vi "Highlight.vi"() -> ()   [LabVIEW 2017]
uses:
  <vilib>/Utility/traverseref.llb/TRef TravTarget.ctl
  user.lib/_NEVSTOP/Communicable State Machine(CSM)/_Polymophic/Add State(s) to Queue By BOOL(Element).vi
  user.lib/_NEVSTOP/Communicable State Machine(CSM)/Communicable State Machine.lvlib
  <vilib>/Utility/traverseref.llb/VI Scripting - Traverse.lvlib
panel:
  in  "Highlight All Scripts":bool
  in  "Highlight Scripts":bool
  out "String":string
  in  "Listbox":i32(listbox)
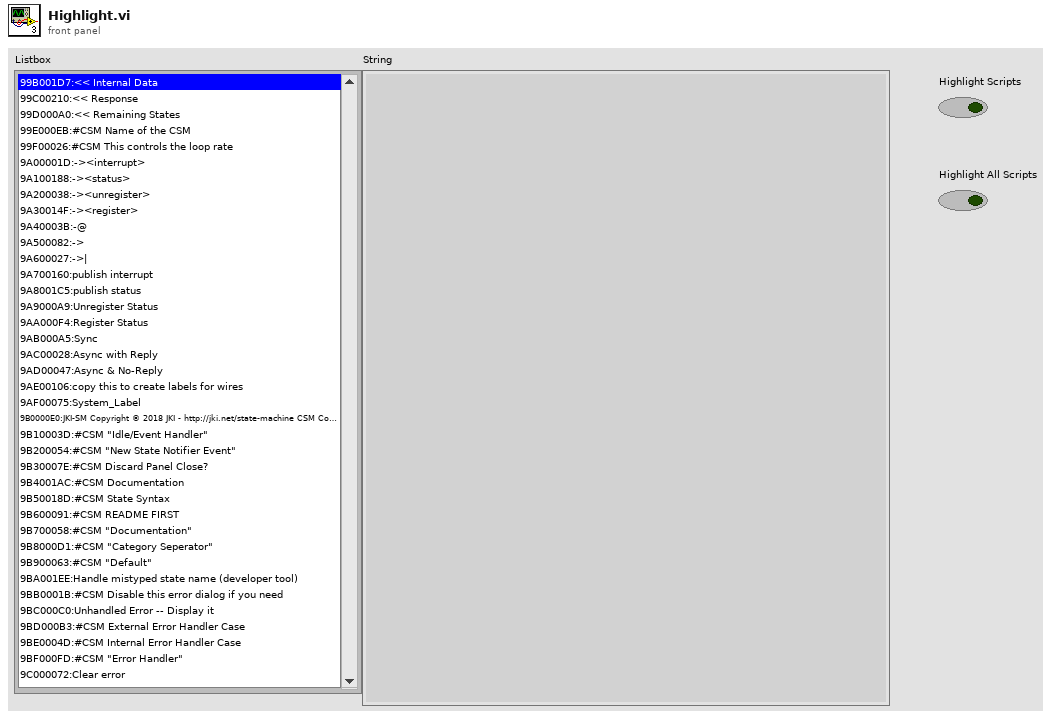
[diagram p1: front panel]
types:
  T1 = enum32{"Invalid", "Standard", "Closed", "Hidden", "Minimized", "Maximized"}
  T2 = enum32{"invalid app kind", "Development System", "Run Time System", "Student Edition", "Embedded LabVIEW", "Evaluation", "Custom"}
  T3 = typedef "TRef TravTarget.ctl" = enum16{"FP", "BD", "Other"}
  T4 = cluster{"Core":cluster{"Current VI Reference":refnum<vi>, "Close Panel on Exit?":bool}, "VI":path, "VIRef":refnum<vi>}
  T5 = cluster{"Current VI Reference":refnum<vi>, "Close Panel on Exit?":bool}
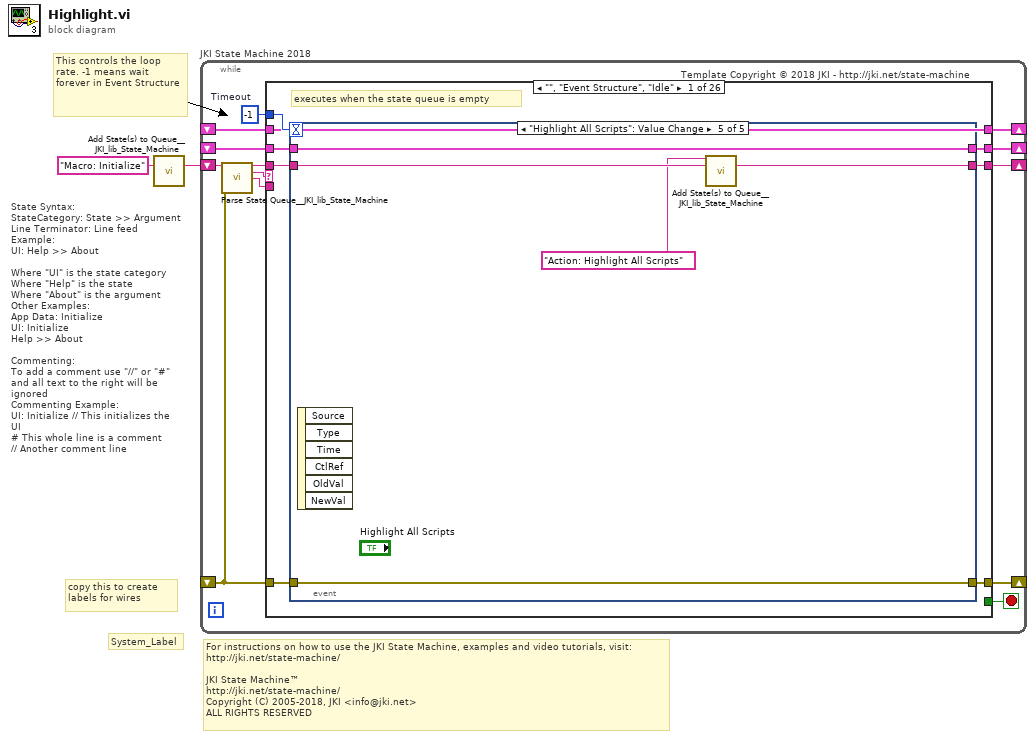
[diagram p0: block diagram]
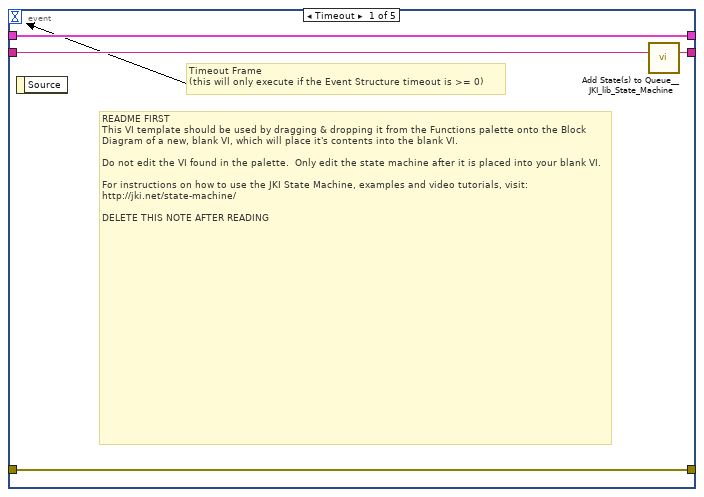
[diagram p2: hidden frame]
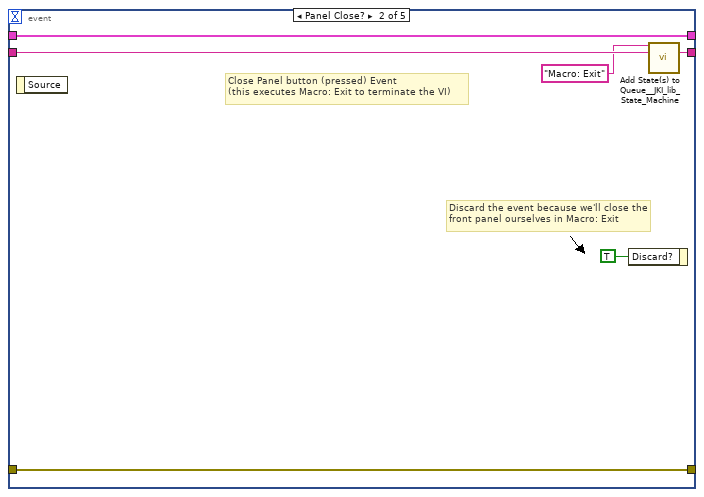
[diagram p3: hidden frame]
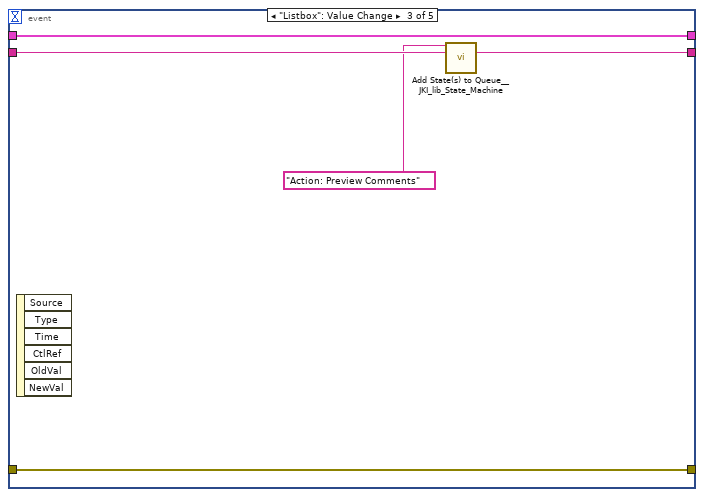
[diagram p4: hidden frame]
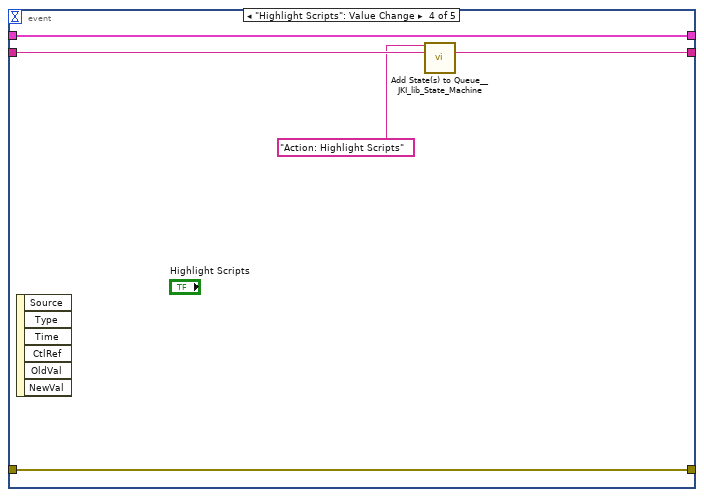
[diagram p5: hidden frame]
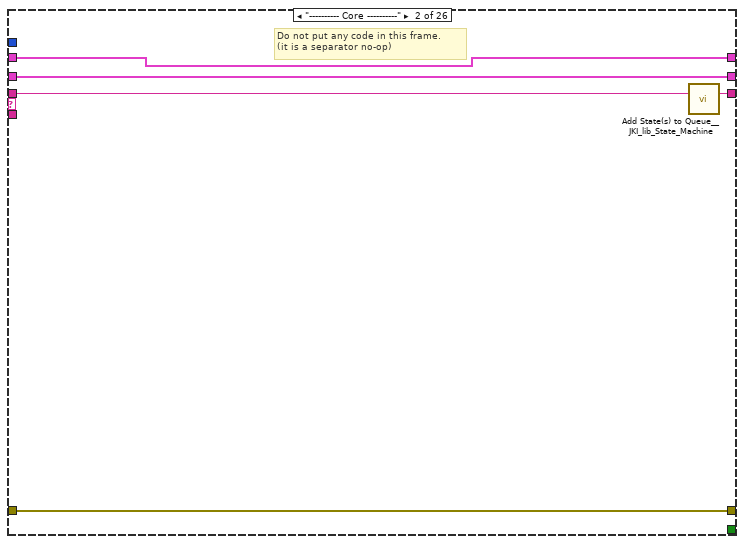
[diagram p6: hidden frame]
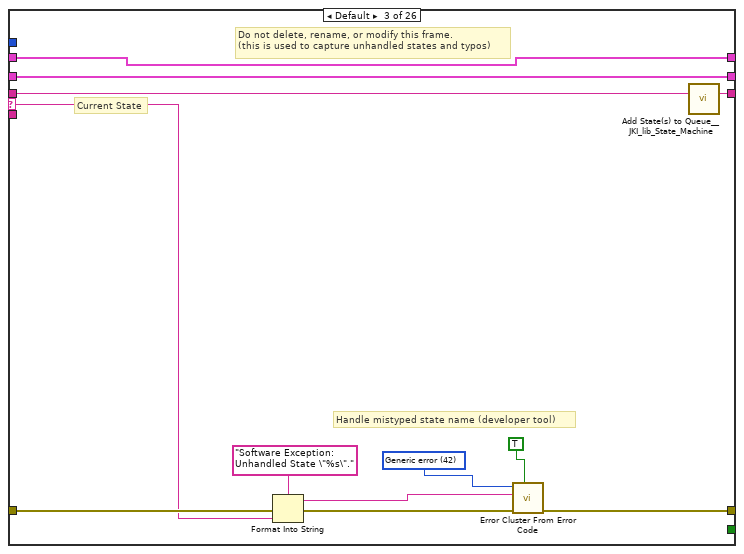
[diagram p7: hidden frame]
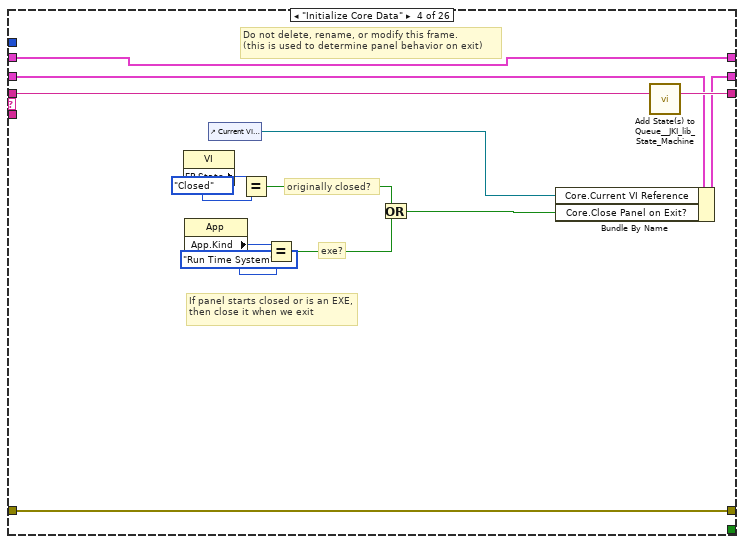
[diagram p8: hidden frame]
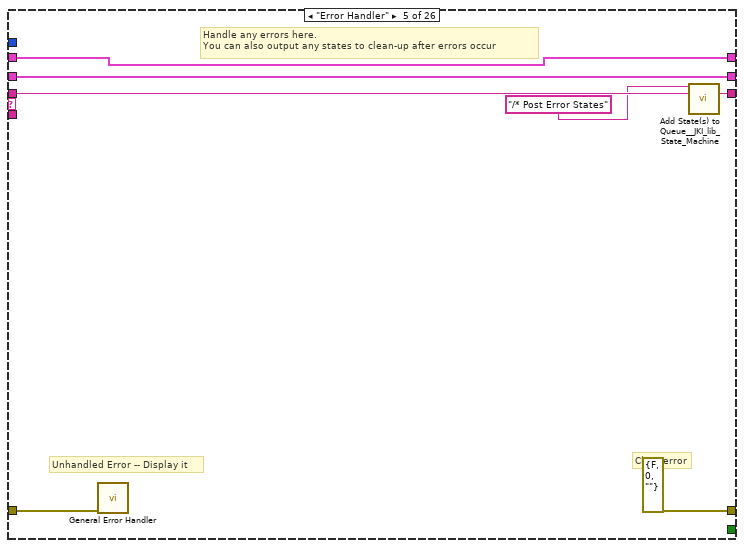
[diagram p9: hidden frame]
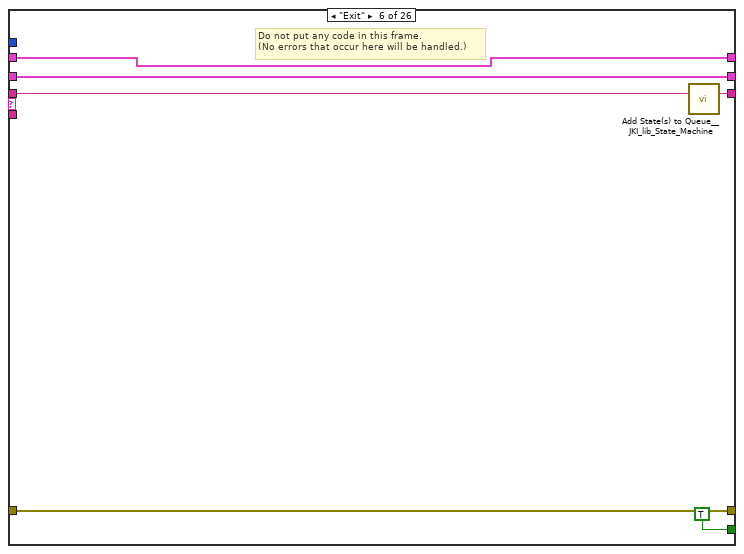
[diagram p10: hidden frame]
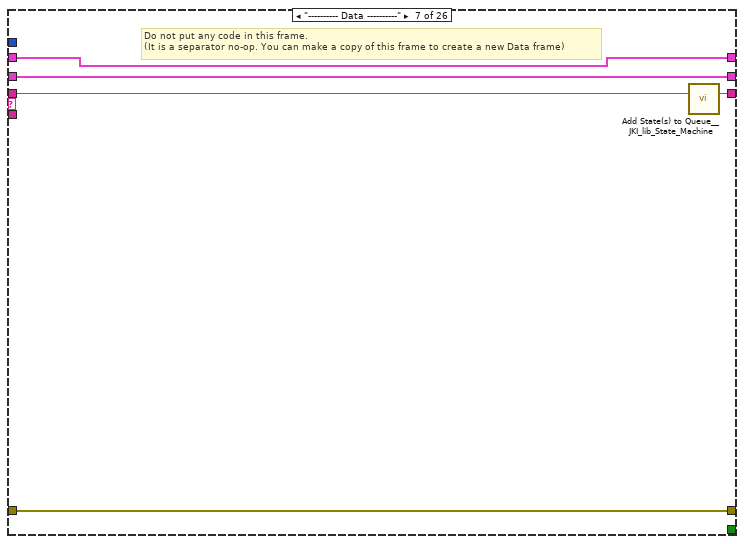
[diagram p11: hidden frame]
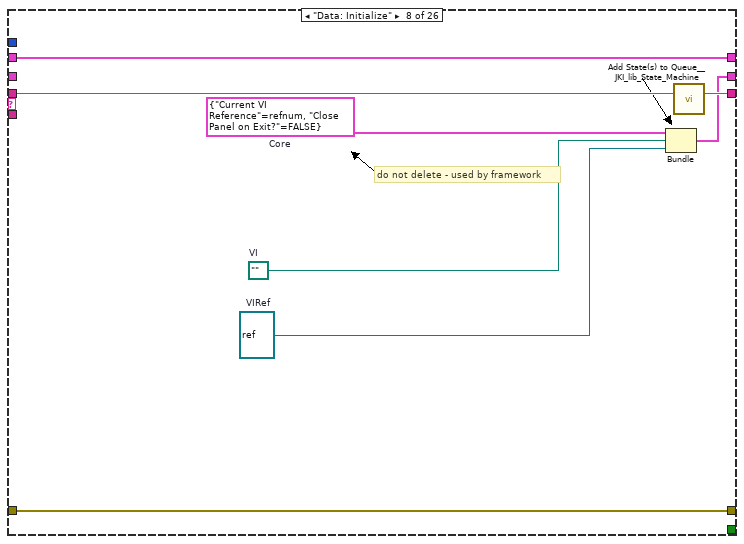
[diagram p12: hidden frame]
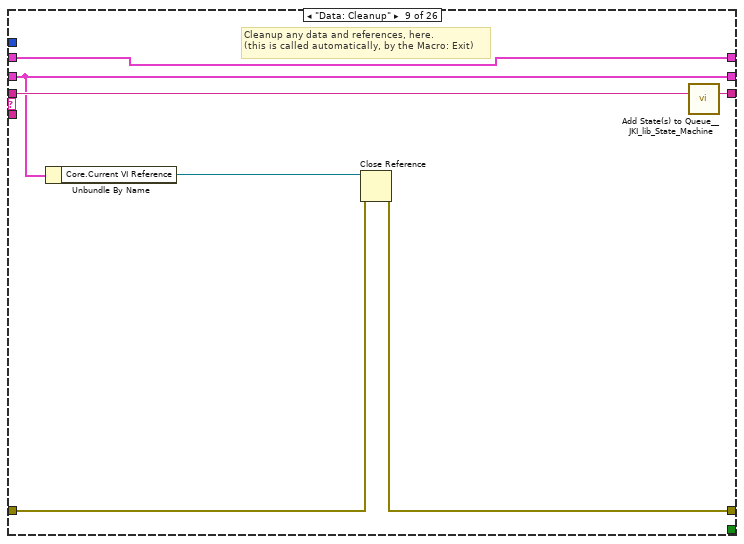
[diagram p13: hidden frame]
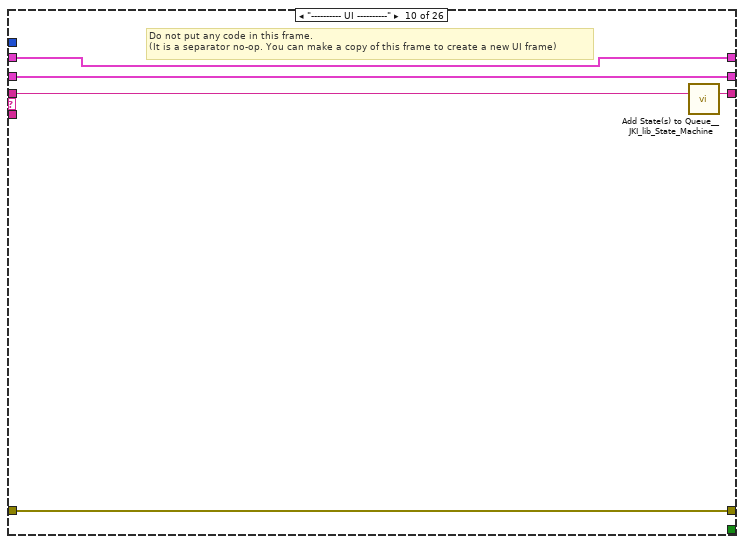
[diagram p14: hidden frame]
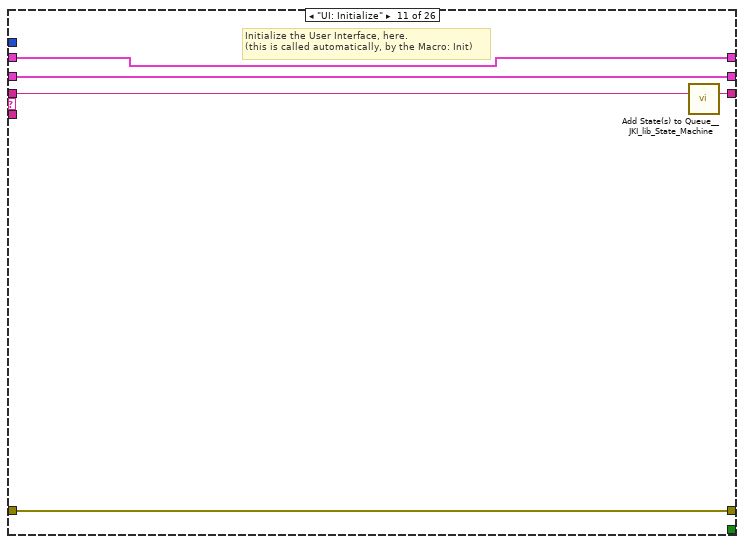
[diagram p15: hidden frame]
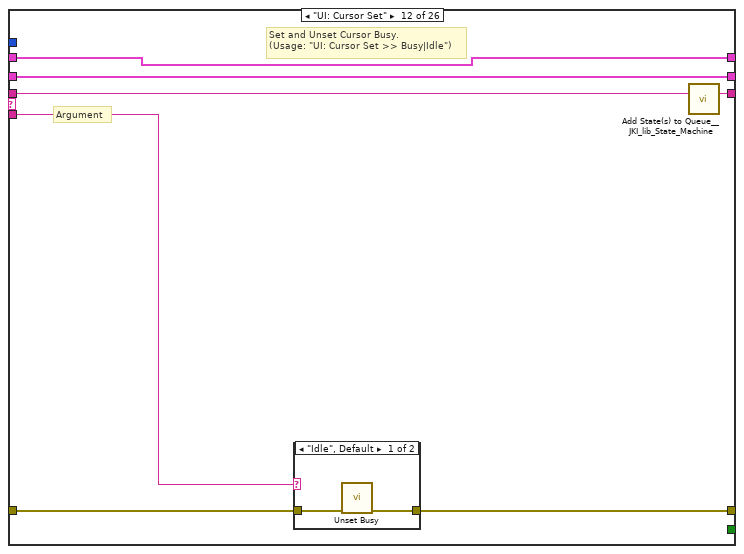
[diagram p16: hidden frame]
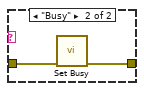
[diagram p17: hidden frame]
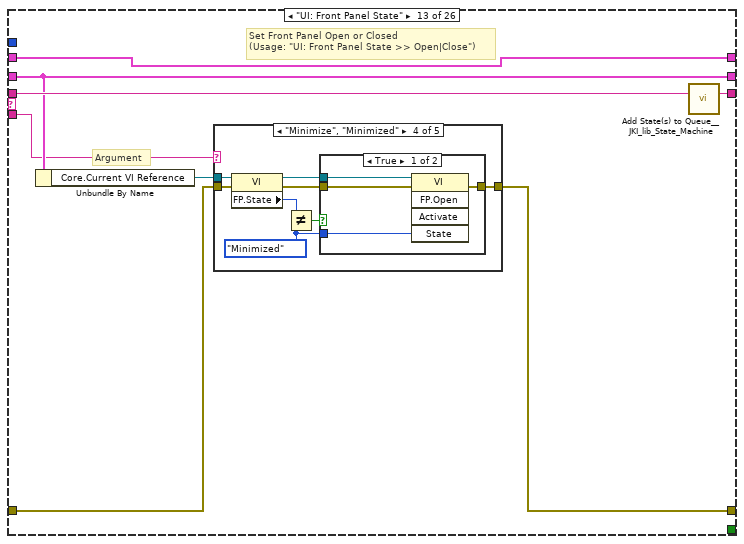
[diagram p18: hidden frame]
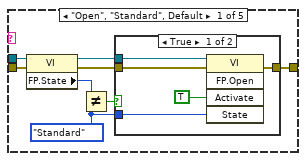
[diagram p19: hidden frame]
diagram:
  # "For instructions on how to use the JKI State Machine, examples and video tutorials, visit:\nhttp://jki.net/state-machine/\n\nJKI State Machine™\nhttp://jki.net/state-machine/\nCopyright (C) 2005-2018, JKI <info@jki.net>\nALL RIGHTS RESERVED"
  # "State Syntax:\nStateCategory: State >> Argument\nLine Terminator: Line feed\nExample:\nUI: Help >> About\n\nWhere \"UI\" is the state category\nWhere \"Help\" is the state\nWhere \"About\" is the argument\nOther Examples:\nApp Data: Initialize\nUI: Initialize\nHelp >> About\n\nCommenting:\nTo add a comment use \"//\" or \"#\" and all text to the right will be ignored\nCommenting Example:\nUI: Initialize // This initializes the UI\n# This whole line is a comment\n// Another comment line"
  # "copy this to create labels for wires"
  # "This controls the loop rate. -1 means wait forever in Event Structure"
  # "System_Label"
  n1 = call <vilib>:"Add State(s) to Queue__JKI_lib_State_Machine.vi"("State(s) in (\"\")"="Macro: Initialize") -> ("States Out"=w1:string)  [unwired: 14 in]
  n2 = while "JKI State Machine 2018" {
    shift-right: [w8] -> _
    shift-left: _ -> [w7]
    shift-right: [w11] -> _
    shift-left: _ -> [w5]
    shift-right: [w10] -> _
    shift-left: w1 -> [w12]
    shift-right: [w4] -> _
    shift-left: _ -> [w3]
    stop <- w9 stop-if-true
    w6 = -1  # Timeout
    # "Template Copyright © 2018 JKI - http://jki.net/state-machine"
    n3 = call <vilib>:"Parse State Queue__JKI_lib_State_Machine.vi"("State Queue"=w12, "Error In (no error)"=w5) -> ("Remaining States"=w14:string, "Current State"=w15:string, "Arguments"=w13:string)  [unwired: 11 in]
    n4 = case shown="\"\", \"Event Structure\", \"Idle\"" w15 {
      selector: w15 -> [_ _ w55 _ _ _ _ _ _ _ _ _ _ _ _ _ _ _ _ _ _ _ _ _ _ _]
      tunnel: w14 -> [w23 w53 w59 w79 w86 w92 w97 w105 w112 w117 w122 w129 w141 w211 w217 w220 w234 w239 w251 w259 w270 w291 w305 w321 w337 w341]
      tunnel: w13 -> [_ _ _ _ _ _ _ _ _ _ _ w124 w135 _ _ _ _ _ _ _ _ _ _ _ _ _]
      tunnel: w7 -> [w21 w50 w57 w72 w83 w90 w94 _ w107 w114 w120 w127 w137 w208 w214 w222 w231 w236 w248 w257 w269 w290 w304 w320 w336 w340]
      tunnel: [w20 w51 w61 w76 errorcluster {"status"=FALSE, "code"=0, "source"=""} ("error out") w89 w95 w102 w108 w115 w119 w125 w138 w209 w215 w223 w232 w237 w249 w260 w271 w292 w306 w322 w327 w339] -> w11
      tunnel: w5 -> [w19 w51 w60 w76 w82 w89 w95 w102 w109 w115 w119 w126 w139 w209 w215 w223 w232 w237 w249 w260 w271 w292 w306 w322 w327 w339]
      tunnel: [w22 w52 w58 w78 w85 w91 w96 w104 w111 w116 w121 w128 w140 w210 w216 w221 w233 w238 w250 w259 w270 w291 w305 w321 w337 w341] -> w10
      tunnel: [_ _ _ _ _ TRUE _ _ _ _ _ _ _ _ _ _ _ _ _ _ _ _ _ _ _ _] -> w9
      tunnel: [w18 w50 w57 w77 w83 w90 w94 w103 w107 w114 w120 w127 w137 w208 w214 w222 w231 w236 w242 w255 w269 w290 w304 w320 w336 w340] -> w8
      tunnel: w6 -> [w17 _ _ _ _ _ _ _ _ _ _ _ _ _ _ _ _ _ _ _ _ _ _ _ _ _]
      tunnel: [w16 w49 w54 w66 w80 w87 w93 w98 w106 w113 w118 w123 w134 w207 w212 w218 w224 w235 w240 cluster{refnum<vi>, "Text.Text":string}[] [] w261 w281 w302 w317 w333 w338] -> w4
      tunnel: w3 -> [w16 w49 w54 w66 w80 w87 w93 w98 w106 w113 w118 w123 w134 w207 w212 w218 w224 w235 w240 _ w262 w282 w302 w317 w333 w338]
      frame "", "Event Structure", "Idle" {
        # "executes when the state queue is empty"
        n5 = event shown="[4] \"Highlight All Scripts\": Value Change" {
          selector: _ -> [_ _ _ _ _]
          dyn-events: _ -> [_ _ _ _ _]
          timeout: w17 -> [_ _ _ _ _]
          tunnel: w23 -> [w27 w33 w35 w40 w45]
          tunnel: [w26 w32 w36 w41 w46] -> w22
          tunnel: w21 -> [w24 w30 w37 w42 w47]
          tunnel: [w25 w31 w38 w43 w48] -> w20
          tunnel: w19 -> [w25 w31 w38 w43 w48]
          tunnel: [w24 w30 w37 w42 w47] -> w18
          event Timeout {
            # "README FIRST\nThis VI template should be used by dragging & dropping it from the Functions palette onto the Block Diagram of a new, blank VI, which will place it's contents into the blank VI.\n\nDo not edit the VI found in the palette.  Only edit the state machine after it is placed into your blank VI.\n\nFor instructions on how to use the JKI State Machine, examples and video tutorials, visit:\nhttp://jki.net/state-machine/\n\nDELETE THIS NOTE AFTER READING"
            # "Timeout Frame\n(this will only execute if the Event Structure timeout is >= 0)"
            n6 = event-data() -> ()  [unwired: 1 in, 1 out]
            n7 = call <vilib>:"Add State(s) to Queue__JKI_lib_State_Machine.vi"("State(s) in (\"\")"=w27) -> ("States Out"=w26:string)  [unwired: 14 in]
          }
          event Panel Close? {
            # "Discard the event because we'll close the front panel ourselves in Macro: Exit"
            # "Close Panel button (pressed) Event\n(this executes Macro: Exit to terminate the VI)"
            n8 = event-data() -> ()  [unwired: 1 in, 1 out]
            n9 = event-data("Discard?"=TRUE) -> ()  [unwired: 1 in, 1 out]
            n10 = call <vilib>:"Add State(s) to Queue__JKI_lib_State_Machine.vi"("State(s) in Front (\"\")"="Macro: Exit", "State(s) in (\"\")"=w33) -> ("States Out"=w32:string)  [unwired: 13 in]
          }
          event "Listbox": Value Change {
            n11 = event-data() -> ()  [unwired: 1 in, 6 out]
            n12 = call <vilib>:"Add State(s) to Queue__JKI_lib_State_Machine.vi"("State(s) in Front (\"\")"="Action: Preview Comments" ("State(s) in Front (\"\")"), "State(s) in (\"\")"=w35) -> ("States Out"=w36:string)  [unwired: 13 in]
          }
          event "Highlight Scripts": Value Change {
            n13 = event-data() -> ()  [unwired: 1 in, 6 out]
            n14 = call <vilib>:"Add State(s) to Queue__JKI_lib_State_Machine.vi"("State(s) in Front (\"\")"="Action: Highlight Scripts" ("State(s) in Front (\"\")"), "State(s) in (\"\")"=w40) -> ("States Out"=w41:string)  [unwired: 13 in]
          }
          event "Highlight All Scripts": Value Change {
            n15 = event-data() -> ()  [unwired: 1 in, 6 out]
            n16 = call <vilib>:"Add State(s) to Queue__JKI_lib_State_Machine.vi"("State(s) in Front (\"\")"="Action: Highlight All Scripts" ("State(s) in Front (\"\")"), "State(s) in (\"\")"=w45) -> ("States Out"=w46:string)  [unwired: 13 in]
          }
        }
      }
      frame "---------- Core ----------" {
        # "Do not put any code in this frame.\n(it is a separator no-op)"
        n17 = call <vilib>:"Add State(s) to Queue__JKI_lib_State_Machine.vi"("State(s) in (\"\")"=w53) -> ("States Out"=w52:string)  [unwired: 14 in]
      }
      frame Default {
        w64 = 42 items=["No error", "Argument error", "Memory is full", "Out of zone", "End of file", "File already open", "Generic file I/O error", "File not found", "File permission error", "Disk is full", "Duplicate path", "Too many files open", "System feature not enabled", "Resource file not found", "Cannot add resource", "Resource not found", "Image not found", "Image memory error", "Pen does not exist", "Config type invalid", "Config token not found", "Config parse error", "Config memory error", "Bad external code format", "Bad external code offset", "External code not present", "Null window", "Destroy window error", "Null menu", "Print aborted", "Bad print record", "Print driver error", "Windows error during printing", "Memory error during printing", "Print dialog error", "Generic print error", "Invalid device refnum", "Device not found", "Device parameter error", "Device unit error", "Cannot open device", "Device call aborted", "Generic error", "Cancelled by user", "Object ID too low", "Object ID too high", "Object not in heap", "Unknown heap", "Unknown object (invalid DefProc)", "Unknown object (DefProc not in table)", "Message out of range", "Invalid (null) method", "Unknown message", "Manager call not supported", "Bad address", "Network operation in progress", "Network operation timed out", "Connection is busy", "Network attribute not supported", "Network error", "Address in use", "System out of memory", "Connection aborted", "Connection refused", "Not connected", "Already connected", "Connection closed", "Initialization error (interapplication manager)", "Bad occurrence", "Wait on unbound occurrence handler", "Occurrence queue overflow", "Datalog type conflict", "Unused", "Unrecognized type (interapplication manager)", "Memory corrupt", "Failed to make temporary DLL", "Old CIN version", "Drag socket not found", "Failed to load drop-object", "Failed to register OLE object", "Failed to release OLE object", "Format specifier type mismatch", "Unknown format specifier", "Too few format specifiers", "Too many format specifiers", "Scan failed", "Newer CIN version", "Error converting to variant", "Runtime menu error", "Password tampered", "Variant attribute not found", "Incompatible variant data type", "Event data is not available", "Event Store is not present", "Occurrence is not found", "Event Queue is not created", "Event info is not available", "Refnum passed is NULL", "Error retrieving Class GUID", "Error retrieving CoClass GUID", "Error retrieving TypeLib GUID.", "Bad built application magic bytes.", "Specific driver is different from the specific driver associated with the Logical Name.", "There is no session opened to the class driver.", "Max Error", "MAX - Error with config objects", "MAX - Error loading configuration", "MAX - Group not supported"]
        # "Current State"
        # "Do not delete, rename, or modify this frame.\n(this is used to capture unhandled states and typos)"
        # "Handle mistyped state name (developer tool)"
        n18 = Format Into String(format string="Software Exception: Unhandled State \"%s\"." ("message"), error in=w60, w55) -> (resulting string=w63:string, error out=w62:errorcluster)  [unwired: 1 in]
        n19 = call <vilib>:"Error Cluster From Error Code.vi"("show call chain? (False)"=TRUE, "error in (no error)"=w62, "error message (\"\")"=w63, "error code (0)"=w64) -> ("error out"=w61:errorcluster)  [unwired: 5 in]
        n20 = call <vilib>:"Add State(s) to Queue__JKI_lib_State_Machine.vi"("State(s) in (\"\")"=w59) -> ("States Out"=w58:string)  [unwired: 14 in]
      }
      frame "Initialize Core Data" {
        # "Do not delete, rename, or modify this frame.\n(this is used to determine panel behavior on exit)"
        # "originally closed?"
        # "exe?"
        # "If panel starts closed or is an EXE, then close it when we exit"
        n21 = property class="VI"() -> ("FP.State"=w69:T1)  [unwired: 2 in, 2 out]
        n22 = property class="App"() -> ("App.Kind"=w75:T2)  [unwired: 2 in, 2 out]
        n23 = control-ref of="Current VI Reference"() -> (w70:refnum<vi>)
        n24 = Equal?(x=w69, y=T1."Closed" ("Front Panel Window:State")) -> (x = y?=w67:bool)
        n25 = Equal?(x=w75, y=T2."Run Time System" ("Application:Kind")) -> (x = y?=w73:bool)
        n26 = Or(x=w67, y=w73) -> (x .or. y?=w71:bool)
        n27 = Bundle By Name(cluster=w72, "Core.Current VI Reference"=w70, "Core.Close Panel on Exit?"=w71) -> (w77:T4)
        n28 = call <vilib>:"Add State(s) to Queue__JKI_lib_State_Machine.vi"("State(s) in (\"\")"=w79) -> ("States Out"=w78:string)  [unwired: 14 in]
      }
      frame "Error Handler" {
        # "Unhandled Error -- Display it"
        # "Handle any errors here.\nYou can also output any states to clean-up after errors occur"
        # "Clear error"
        n29 = call <vilib>:"General Error Handler.vi"("error in (no error)"=w82) -> ()  [unwired: 10 in, 5 out]
        n30 = call <vilib>:"Add State(s) to Queue__JKI_lib_State_Machine.vi"("State(s) in Front (\"\")"="/* Post Error States", "State(s) in (\"\")"=w86) -> ("States Out"=w85:string)  [unwired: 13 in]
      }
      frame "Exit" {
        # "Do not put any code in this frame.\n(No errors that occur here will be handled.)"
        n31 = call <vilib>:"Add State(s) to Queue__JKI_lib_State_Machine.vi"("State(s) in (\"\")"=w92) -> ("States Out"=w91:string)  [unwired: 14 in]
      }
      frame "---------- Data ----------" {
        # "Do not put any code in this frame.\n(It is a separator no-op. You can make a copy of this frame to create a new Data frame)"
        n32 = call <vilib>:"Add State(s) to Queue__JKI_lib_State_Machine.vi"("State(s) in (\"\")"=w97) -> ("States Out"=w96:string)  [unwired: 14 in]
      }
      frame "Data: Initialize" {
        w99 = refnum<vi> refnum  # VIRef
        w100 = T5 {"Current VI Reference"=refnum, "Close Panel on Exit?"=FALSE}  # Core
        w101 = path ""  # VI
        # "do not delete - used by framework"
        n33 = Bundle("Core"=w100, "VI"=w101, "VIRef"=w99) -> (w103:T4)  [unwired: 1 in]
        n34 = call <vilib>:"Add State(s) to Queue__JKI_lib_State_Machine.vi"("State(s) in (\"\")"=w105) -> ("States Out"=w104:string)  [unwired: 14 in]
      }
      frame "Data: Cleanup" {
        # "Cleanup any data and references, here.\n(this is called automatically, by the Macro: Exit)"
        n35 = Unbundle By Name(w107) -> ("Core.Current VI Reference"=w110:refnum<vi>)
        n36 = Close Reference(reference=w110, error in (no error)=w109) -> (error out=w108:errorcluster)
        n37 = call <vilib>:"Add State(s) to Queue__JKI_lib_State_Machine.vi"("State(s) in (\"\")"=w112) -> ("States Out"=w111:string)  [unwired: 14 in]
      }
      frame "---------- UI ----------" {
        # "Do not put any code in this frame.\n(It is a separator no-op. You can make a copy of this frame to create a new UI frame)"
        n38 = call <vilib>:"Add State(s) to Queue__JKI_lib_State_Machine.vi"("State(s) in (\"\")"=w117) -> ("States Out"=w116:string)  [unwired: 14 in]
      }
      frame "UI: Initialize" {
        # "Initialize the User Interface, here.\n(this is called automatically, by the Macro: Init)"
        n39 = call <vilib>:"Add State(s) to Queue__JKI_lib_State_Machine.vi"("State(s) in (\"\")"=w122) -> ("States Out"=w121:string)  [unwired: 14 in]
      }
      frame "UI: Cursor Set" {
        # "Argument"
        # "Set and Unset Cursor Busy.\n(Usage: \"UI: Cursor Set >> Busy|Idle\")"
        n40 = case shown="\"Idle\", Default" w124 {
          tunnel: w126 -> [w131 w133]
          tunnel: [w130 w132] -> w125
          frame "Idle", Default {
            n41 = call <vilib>:"Unset Busy.vi"("error in (no error)"=w131) -> ("error out"=w130:errorcluster)  [unwired: 10 in]
          }
          frame "Busy" {
            n42 = call <vilib>:"Set Busy.vi"("error in (no error)"=w133) -> ("error out"=w132:errorcluster)  [unwired: 9 in, 1 out]
          }
        }
        n43 = call <vilib>:"Add State(s) to Queue__JKI_lib_State_Machine.vi"("State(s) in (\"\")"=w129) -> ("States Out"=w128:string)  [unwired: 14 in]
      }
      frame "UI: Front Panel State" {
        # "Argument"
        # "Set Front Panel Open or Closed\n(Usage: \"UI: Front Panel State >> Open|Close\")"
        n44 = Unbundle By Name(w137) -> ("Core.Current VI Reference"=w136:refnum<vi>)
        n45 = case shown="\"Minimize\", \"Minimized\"" w135 {
          tunnel: w139 -> [w147 w162 w173 w186 w199]
          tunnel: [w149 w163 w175 w188 w201] -> w138
          tunnel: w136 -> [w148 w160 w174 w187 w200]
          frame "Open", "Standard", Default {
            w142 = T1."Standard" ("State")
            n46 = property class="VI"(reference=w148, error in=w147) -> (reference out=w145:refnum<vi>, error out=w146:errorcluster, "FP.State"=w144:T1)
            n47 = Not Equal?(x=w144, y=w142) -> (x != y?=w143:bool)
            n48 = case shown="True" w143 {
              tunnel: [w153 w155] -> w149
              tunnel: w146 -> [w152 w155]
              tunnel: w145 -> [w151 _]
              tunnel: w142 -> [w150 _]
              frame True {
                n49 = invoke class="VI" method="FP.Open"(reference=w151, error in=w152, "Activate"=TRUE, "State"=w150) -> (error out=w153:errorcluster)  [unwired: 1 in, 4 out]
              }
              frame False {
              }
            }
          }
          frame "Close", "Closed" {
            n50 = property class="VI"(reference=w160, error in=w162) -> (reference out=w159:refnum<vi>, error out=w161:errorcluster, "FP.State"=w157:T1)
            n51 = Not Equal?(x=w157, y=T1."Closed" ("Front Panel Window:State")) -> (x != y?=w156:bool)
            n52 = case shown="True" w156 {
              tunnel: [w164 w167] -> w163
              tunnel: w161 -> [w164 w166]
              tunnel: w159 -> [_ w165]
              frame False {
              }
              frame True {
                n53 = invoke class="VI" method="FP.Close"(reference=w165, error in=w166) -> (error out=w167:errorcluster)  [unwired: 1 in, 2 out]
              }
            }
          }
          frame "Hidden", "Hide" {
            w168 = T1."Hidden" ("State")
            n54 = property class="VI"(reference=w174, error in=w173) -> (reference out=w171:refnum<vi>, error out=w172:errorcluster, "FP.State"=w170:T1)
            n55 = Not Equal?(x=w170, y=w168) -> (x != y?=w169:bool)
            n56 = case shown="True" w169 {
              tunnel: [w179 w180] -> w175
              tunnel: w172 -> [w178 w180]
              tunnel: w171 -> [w177 _]
              tunnel: w168 -> [w176 _]
              frame True {
                n57 = invoke class="VI" method="FP.Open"(reference=w177, error in=w178, "State"=w176) -> (error out=w179:errorcluster)  [unwired: 2 in, 4 out]
              }
              frame False {
              }
            }
          }
          frame "Minimize", "Minimized" {
            w181 = T1."Minimized" ("State")
            n58 = property class="VI"(reference=w187, error in=w186) -> (reference out=w184:refnum<vi>, error out=w185:errorcluster, "FP.State"=w183:T1)
            n59 = Not Equal?(x=w183, y=w181) -> (x != y?=w182:bool)
            n60 = case shown="True" w182 {
              tunnel: [w192 w193] -> w188
              tunnel: w185 -> [w191 w193]
              tunnel: w184 -> [w190 _]
              tunnel: w181 -> [w189 _]
              frame True {
                n61 = invoke class="VI" method="FP.Open"(reference=w190, error in=w191, "State"=w189) -> (error out=w192:errorcluster)  [unwired: 2 in, 4 out]
              }
              frame False {
              }
            }
          }
          frame "Maximize", "Maximized" {
            w194 = T1."Maximized" ("State")
            n62 = property class="VI"(reference=w200, error in=w199) -> (reference out=w197:refnum<vi>, error out=w198:errorcluster, "FP.State"=w196:T1)
            n63 = Not Equal?(x=w196, y=w194) -> (x != y?=w195:bool)
            n64 = case shown="True" w195 {
              tunnel: [w205 w206] -> w201
              tunnel: w198 -> [w204 w206]
              tunnel: w197 -> [w203 _]
              tunnel: w194 -> [w202 _]
              frame True {
                n65 = invoke class="VI" method="FP.Open"(reference=w203, error in=w204, "State"=w202) -> (error out=w205:errorcluster)  [unwired: 2 in, 4 out]
              }
              frame False {
              }
            }
          }
        }
        n66 = call <vilib>:"Add State(s) to Queue__JKI_lib_State_Machine.vi"("State(s) in (\"\")"=w141) -> ("States Out"=w140:string)  [unwired: 14 in]
      }
      frame "---------- Macro ----------" {
        # "Do not put any code in this frame.\n(It is a separator no-op. You can make a copy of this frame to create a new Macro frame)"
        n67 = call <vilib>:"Add State(s) to Queue__JKI_lib_State_Machine.vi"("State(s) in (\"\")"=w211) -> ("States Out"=w210:string)  [unwired: 14 in]
      }
      frame "Macro: Initialize" {
        w213 = "Data: Initialize\nInitialize Core Data\nUI: Initialize\nUI: Front Panel State >> Open\n//\nAction: Load VI"  # Data: Initialize Initialize Core Data UI: Initialize UI: Front Panel State >> Open // Action: Load VI
        # "Initialization Macro\n(This is called once, when the VI starts)"
        n68 = call <vilib>:"Add State(s) to Queue__JKI_lib_State_Machine.vi"("State(s) in Front (\"\")"=w213, "State(s) in (\"\")"=w217) -> ("States Out"=w216:string)  [unwired: 13 in]
      }
      frame "Macro: Script" {
        n69 = call <vilib>:"Add State(s) to Queue__JKI_lib_State_Machine.vi"("State(s) in Front (\"\")"="Action: OpenVI\nAction: Load Text Decor\nAction: Load StringConstant\nAction: Update UI" ("State(s) in Front (\"\")"), "State(s) in (\"\")"=w220) -> ("States Out"=w221:string)  [unwired: 13 in]
      }
      frame "Macro: Exit" {
        # "Exit Macro\n(This is called once, when the VI exits)"
        n70 = Unbundle By Name(w231) -> ("Core.Close Panel on Exit?"=w230:bool)
        n71 = Select(t="UI: Front Panel State >> Close", s=w230, f="") -> (s? t:f=w227:string)
        n72 = call <vilib>:"Add State(s) to Queue__JKI_lib_State_Machine.vi"("State(s) in (\"\")"=w227, "State(s) at Back (\"\")"="Data: Cleanup\nExit") -> ("States Out"=w225:string)  [unwired: 13 in]
        n73 = call <vilib>:"Add State(s) to Queue__JKI_lib_State_Machine.vi"("State(s) in Front (\"\")"=w225, "State(s) in (\"\")"=w234) -> ("States Out"=w233:string)  [unwired: 13 in]
      }
      frame "---------- Action ----------" {
        # "Template Separator\n(You can make a copy of, or modify, this frame)"
        n74 = call <vilib>:"Add State(s) to Queue__JKI_lib_State_Machine.vi"("State(s) in (\"\")"=w239) -> ("States Out"=w238:string)  [unwired: 14 in]
      }
      frame "Action: Load VI" {
        n75 = call "File Dialog"("pattern (all files)"="*.vi") -> ("selected path"=w241:path, "error out"=w246:errorcluster)  [unwired: 11 in, 2 out]
        n76 = Not(x=w246) -> (.not. x?=w245:bool)
        n77 = Bundle By Name(cluster=w248, "VI"=w241) -> (w242:T4)
        n78 = call-poly "Add State(s) to Queue By BOOL++.vi"("False(\"\")"="Macro: Exit" ("pattern (all files)"), "TRUE(\"\")"="Macro: Script" ("pattern (all files)"), "Bool"=w245, "State Queue(\"\")"=w251) -> ("State Queue Out"=w250:string)  [unwired: 7 in]
      }
      frame "Action: OpenVI" {
        n79 = Unbundle By Name(w257) -> ("VI"=w256:path)
        n80 = Open VI Reference(vi path=w256, options=2) -> (vi reference=w253:refnum<vi>)  [unwired: 4 in, 1 out]
        n81 = invoke class="VI" method="FP.Open"(reference=w253) -> (reference out=w254:refnum<vi>)  [unwired: 4 in, 4 out]
        n82 = Bundle By Name(cluster=w257, "VIRef"=w254) -> (w255:T4)
      }
      frame "Action: Load Text Decor" {
        n83 = Unbundle By Name(w269) -> ("VIRef"=w263:refnum<vi>)
        n84 = call <vilib>:"Traverse for GObjects.vi"("Traverse Target"=TRef_TravTarget."BD", "Class Name"="Text", "VI Refnum"=w263) -> ("error out"=w264:errorcluster, "References"=w266:refnum<vi>[])  [unwired: 5 in, 2 out]
        n85 = for {
          tunnel: w266 -> [w272] mode=indexing
          tunnel: w264 -> [w280]
          tunnel: [w277] -> w265 mode=indexing if=w275
          n86 = To More Specific Class(target class=refnum<vi> refnum ("reference out"), reference=w272, error in=w280) -> (specific class reference=w279:refnum<vi>, error out=w278:errorcluster)
          n87 = property class="Txt"(reference=w279, error in=w278) -> (error out=w276:errorcluster, "Text"=w274:string)  [unwired: 1 out]
          n88 = Not(x=w276) -> (.not. x?=w275:bool)
          n89 = Bundle(w272, "Text"=w274) -> (w277:cluster{refnum<vi>, "Text":string})  [unwired: 1 in]
        }
        n90 = Build Array (concatenate)(w262, w265) -> (w261:cluster{refnum<vi>, "Text":string}[])
      }
      frame "Action: Load StringConstant" {
        n91 = Unbundle By Name(w290) -> ("VIRef"=w284:refnum<vi>)
        n92 = call <vilib>:"Traverse for GObjects.vi"("Traverse Target"=TRef_TravTarget."BD", "Class Name"="StringConstant", "VI Refnum"=w284) -> ("error out"=w285:errorcluster, "References"=w287:refnum<vi>[])  [unwired: 5 in, 2 out]
        n93 = for {
          tunnel: w287 -> [w293] mode=indexing
          tunnel: w285 -> [w301]
          tunnel: [w298] -> w286 mode=indexing if=w296
          tunnel: refnum<vi> refnum ("reference out") -> [w294]
          n94 = To More Specific Class(target class=w294, reference=w293, error in=w301) -> (specific class reference=w300:refnum<vi>, error out=w299:errorcluster)
          n95 = property class="StrCnst"(reference=w300, error in=w299) -> (error out=w297:errorcluster, "Text.Text"=w295:string)  [unwired: 1 out]
          n96 = Not(x=w297) -> (.not. x?=w296:bool)
          n97 = Bundle(w293, "Text.Text"=w295) -> (w298:cluster{refnum<vi>, "Text.Text":string})  [unwired: 1 in]
        }
        n98 = Build Array (concatenate)(w282, w286) -> (w281:cluster{refnum<vi>, "Text.Text":string}[])
      }
      frame "Action: Update UI" {
        n99 = for {
          tunnel: w302 -> [w315] mode=indexing
          tunnel: [w307] -> w303 mode=indexing
          w309 = u32 0  # U32
          n100 = Unbundle(w315) -> (w311:refnum<vi>, "Text.Text"=w314:string)
          n101 = call "CSM - Break Down Multiple States String.vi"("States"=w314) -> ("Multiple States"=w313:string[])  [unwired: 10 in]
          n102 = Type Cast(type=w309, x=w311) -> (*(type *) &x=w308:u32)
          n103 = Index Array(array=w313) -> (element=w312:string)  [unwired: 1 in]
          n104 = Format Into String(format string="%x:%s", w308, w312) -> (resulting string=w307:string)  [unwired: 2 in, 1 out]
        }
        n105 = property on="Listbox" class="LstBox (strict)"("Item Names"=w303) -> ()  [unwired: 2 in, 2 out]
      }
      frame "Action: Preview Comments" {
        n106 = Index Array(array=w317, index="Listbox") -> (element=w318:cluster{refnum<vi>, "Text.Text":string})
        n107 = Unbundle(w318) -> ("Text.Text"=→"String":string)  [unwired: 1 out]
      }
      frame "Action: Highlight Scripts" {
        n108 = local read "Listbox"() -> (w335:i32)
        n109 = Index Array(array=w333, index=w335) -> (element=w334:cluster{refnum<vi>, "Text.Text":string})
        n110 = Unbundle(w334) -> (w329:refnum<vi>)  [unwired: 1 out]
        n111 = To More Specific Class(target class=refnum<vi> refnum ("reference out"), reference=w329) -> (specific class reference=w331:refnum<vi>, error out=w324:errorcluster)  [unwired: 1 in]
        n112 = To More Specific Class(target class=refnum<vi> refnum ("reference out"), reference=w329) -> (specific class reference=w328:refnum<vi>, error out=w323:errorcluster)  [unwired: 1 in]
        n113 = call "_Highlight CSM Scripts(TextDecor).vi"("error in (no error)"=w324, "reference out 2"=w331) -> ("error out"=w325:errorcluster)  [unwired: 9 in]
        n114 = call "_Highlight CSM Scripts(StringConstant).vi"("error in (no error)"=w323, "reference out"=w328) -> ("error out"=w326:errorcluster)  [unwired: 9 in]
        n115 = call <vilib>:"Clear Errors.vi"("error in (no error)"=w325) -> ()  [unwired: 5 in, 2 out]
        n116 = call <vilib>:"Clear Errors.vi"("error in (no error)"=w326) -> ()  [unwired: 5 in, 2 out]
      }
      frame "Action: Highlight All Scripts" {
        n117 = for {
          tunnel: w338 -> [w342] mode=indexing
          n118 = Unbundle(w342) -> (w348:refnum<vi>)  [unwired: 1 out]
          n119 = To More Specific Class(target class=refnum<vi> refnum ("reference out"), reference=w348) -> (specific class reference=w350:refnum<vi>, error out=w344:errorcluster)  [unwired: 1 in]
          n120 = To More Specific Class(target class=refnum<vi> refnum ("reference out"), reference=w348) -> (specific class reference=w347:refnum<vi>, error out=w343:errorcluster)  [unwired: 1 in]
          n121 = call "_Highlight CSM Scripts(TextDecor).vi"("error in (no error)"=w344, "reference out 2"=w350) -> ("error out"=w345:errorcluster)  [unwired: 9 in]
          n122 = call "_Highlight CSM Scripts(StringConstant).vi"("error in (no error)"=w343, "reference out"=w347) -> ("error out"=w346:errorcluster)  [unwired: 9 in]
          n123 = call <vilib>:"Clear Errors.vi"("error in (no error)"=w345) -> ()  [unwired: 5 in, 2 out]
          n124 = call <vilib>:"Clear Errors.vi"("error in (no error)"=w346) -> ()  [unwired: 5 in, 2 out]
        }
      }
    }
  }
